vi "Connect_to_uArm.vi"(8 "error in":errorcluster, 10 "full read buffer in":string, 11 "Machine In":refnum<visa-resource-name>="ASRL1::INSTR") -> (0 "error out":errorcluster, 2 "full read buffer out":string, 3 "Machine Out":refnum<visa-resource-name>)   [LabVIEW 2017]
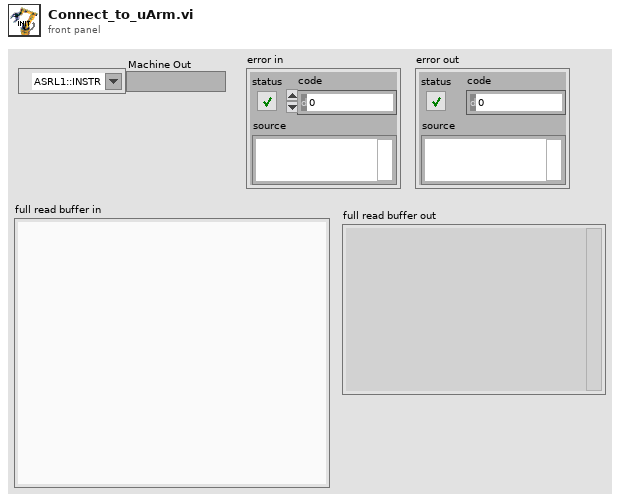
[diagram p1: front panel]
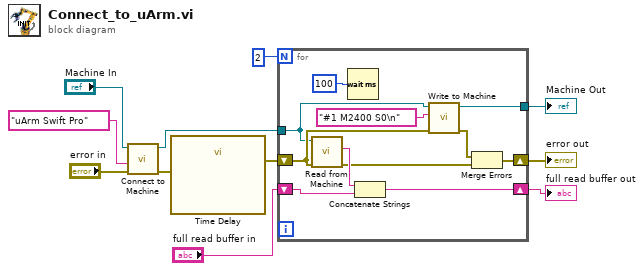
[diagram p0: block diagram]
diagram:
  n1 = call "Connect to Machine .vi"("error in"="error in", "Firmware"="uArm Swift Pro", "Machine In"="Machine In") -> ("error out"=w10:errorcluster, "Machine Out"=w2:refnum<visa-resource-name>)  [unwired: 6 in, 1 out]
  n2 = call "Time Delay"("error in (no error)"=w10) -> ("error out"=w6:errorcluster)  [unwired: 10 in]
  n3 = for {
    N: 2 -> [_]
    tunnel: w2 -> [w15]
    shift-right: [w14] -> w4
    shift-left: w6 -> [w16]
    tunnel: [w13] -> w5
    shift-right: [w12] -> w3
    shift-left: "full read buffer in" -> [w17]
    n4 = call "Read from Machine.vi"("error in (no error)"=w16, "Machine In"=w15) -> ("error out"=w20:errorcluster, "read buffer"=w21:string)  [unwired: 7 in, 1 out]
    n5 = Wait (ms)(milliseconds to wait=u32 100) -> ()  [unwired: 1 out]
    n6 = Concatenate Strings(w21, w17) -> (w12:string)
    n7 = call "Write to Machine .vi"("error in (no error)"=w16, "G-Code String In"="#1 M2400 S0\n", "Machine In"=w15) -> ("error out"=w19:errorcluster, "Machine Out"=w13:refnum<visa-resource-name>)  [unwired: 7 in]
    n8 = Merge Errors(w19, w20) -> (w14:errorcluster)
  }
  "error out" <- w4
  "Machine Out" <- w5
  "full read buffer out" <- w3
